vi "Simple Shared Variable and Event Monitor.vi"() -> ()   [LabVIEW 2015]
doc: "This example demonstrates how to build a variable and event monitor using the shared variable Event structure support. \nRefer to the readme.html file in the <b>Project Documentation</b> folder of the project tree for more information about this example."
uses:
  Instance           1 30Saved   Simple Process Monitor .vi
  <vilib>/lvdsc/NI_DSC.lvlib
panel:
  in  "Stop?":bool
  in  "Refresh Variable List":bool
  in  "Delete Variable Button":bool
  in  "Variable List":i32(listbox)=-1
  in  "Delete Process Button":bool
  in  "Deployed Processes":i32(listbox)=-1
  in  "System Events":i32(listbox)=-1
  out "error out":errorcluster
  in  "error in (no error)":errorcluster
  # "LabVIEW DSC Module Example: \nSimple Shared Variable and Event Monitor"
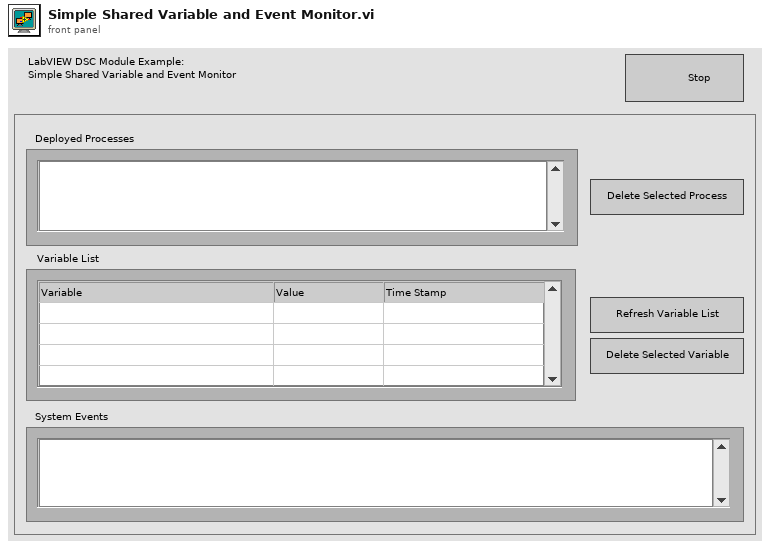
[diagram p1: front panel]
types:
  T1 = enum16{"No Value", "Custom", "Double", "Boolean", "U32", "String", "DBL Array", "I32 Array", "I32", "SGL Array", "SGL", "I8", "U8", "I16", "U16", "I64", "U64", "DBL Waveform", "I16 Waveform", "Boolean Array", "I8 Array", "U8 Array", "I16 Array", "U16 Array", "U32 Array", "I64 Array", "U64 Array", "DBL Waveform Array", "I16 Waveform Array"}
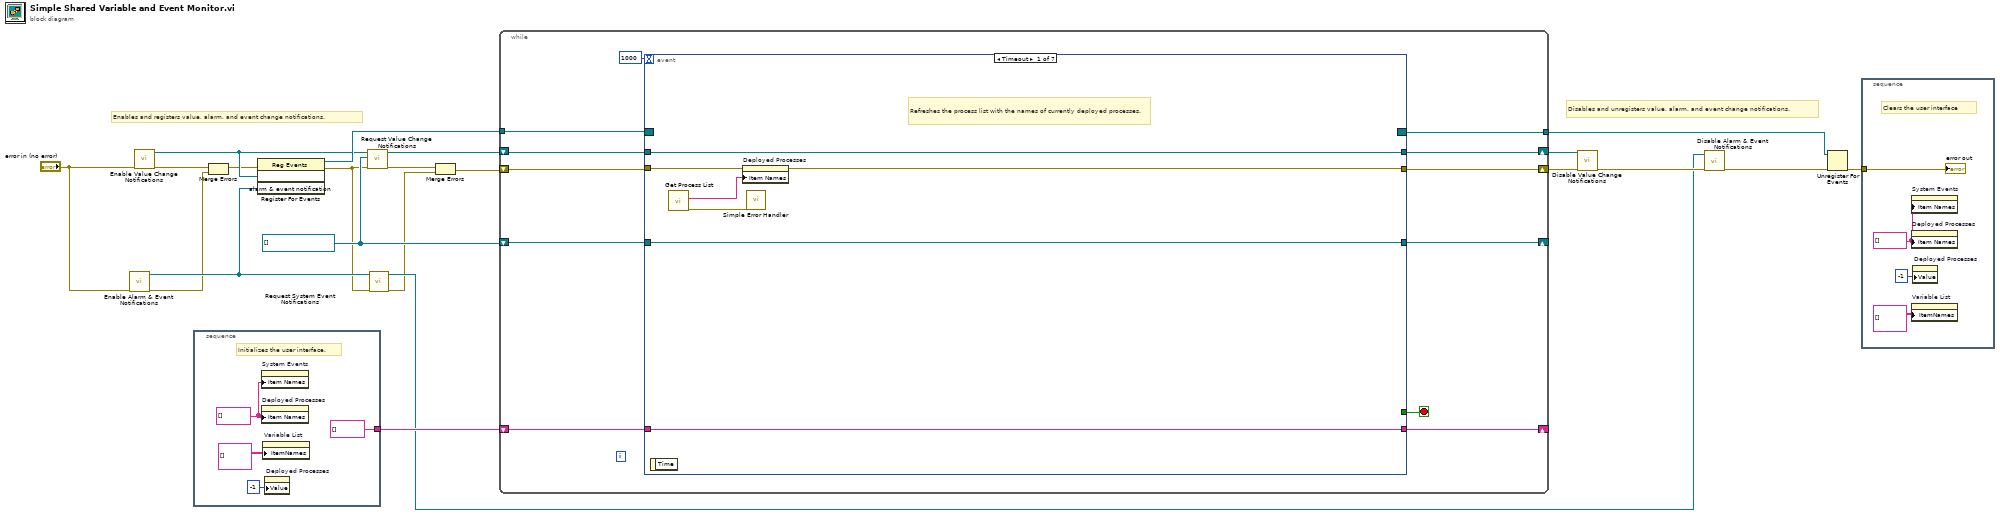
[diagram p0: block diagram]
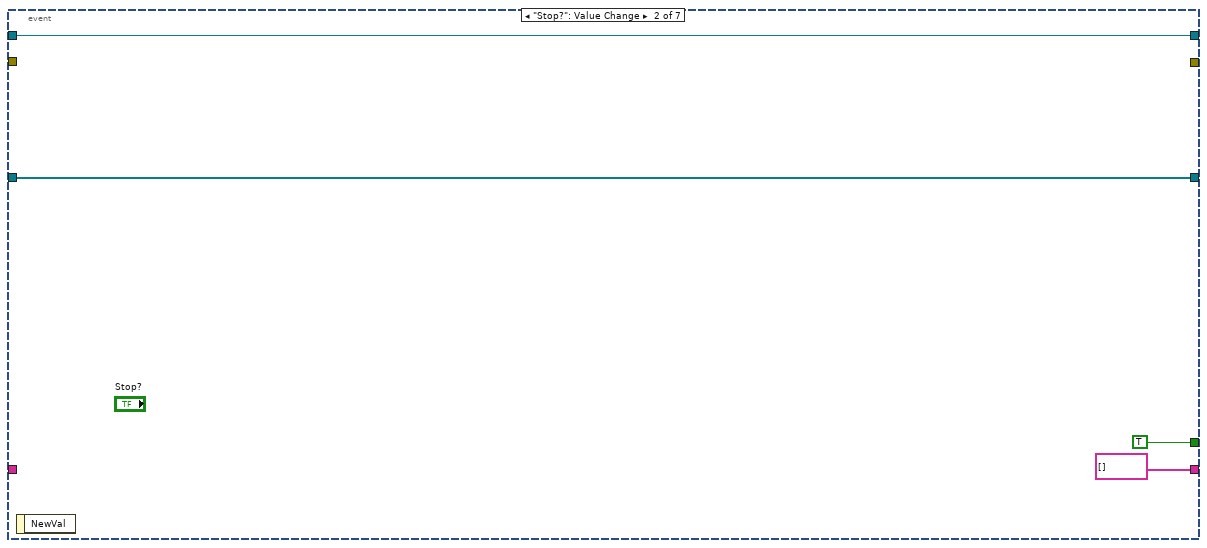
[diagram p2: hidden frame]
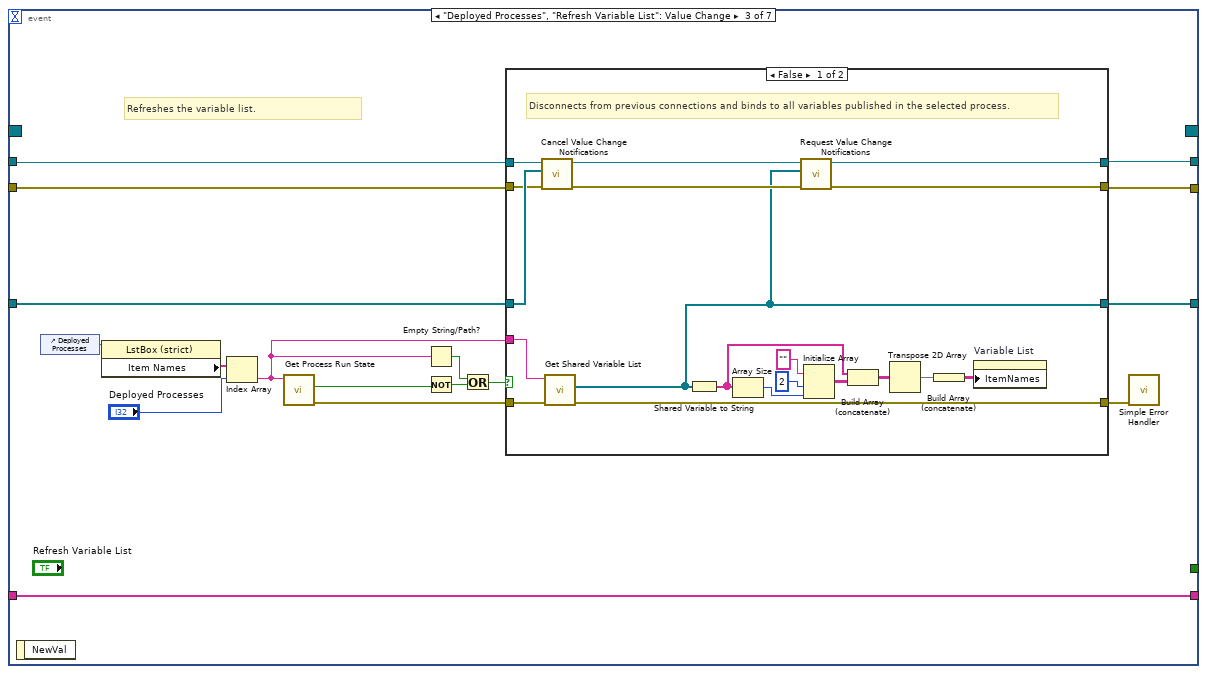
[diagram p3: hidden frame]
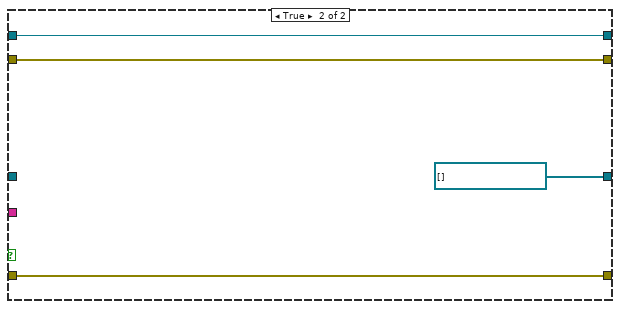
[diagram p4: hidden frame]
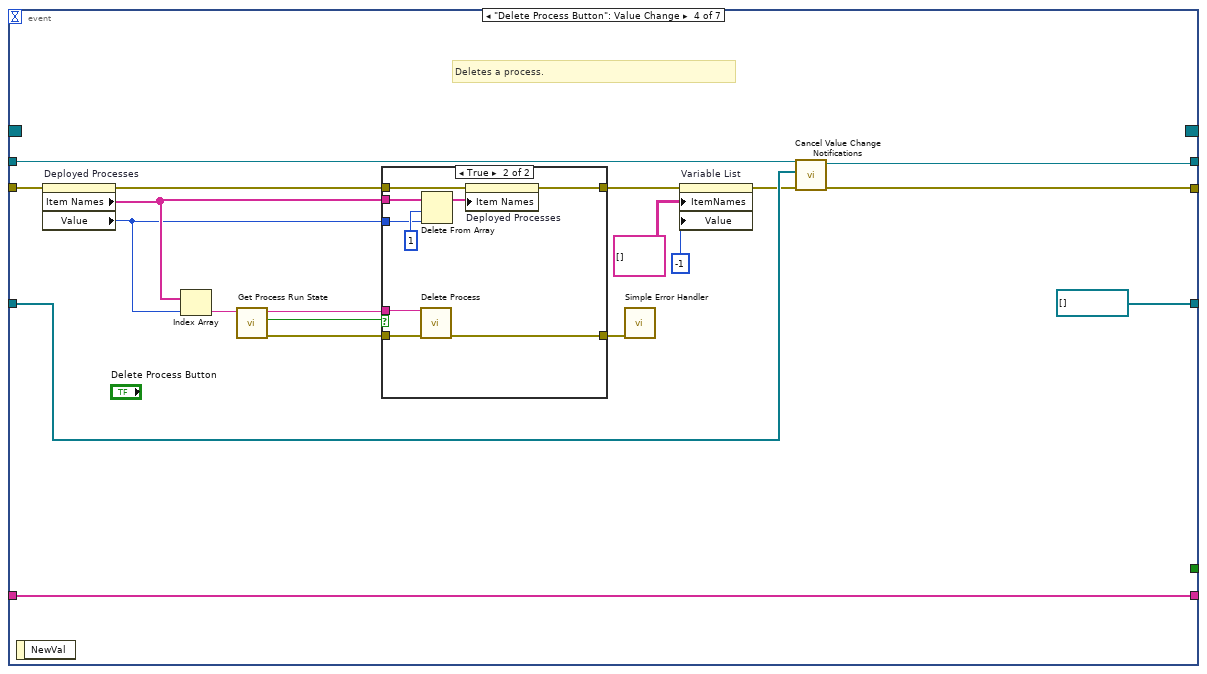
[diagram p5: hidden frame]
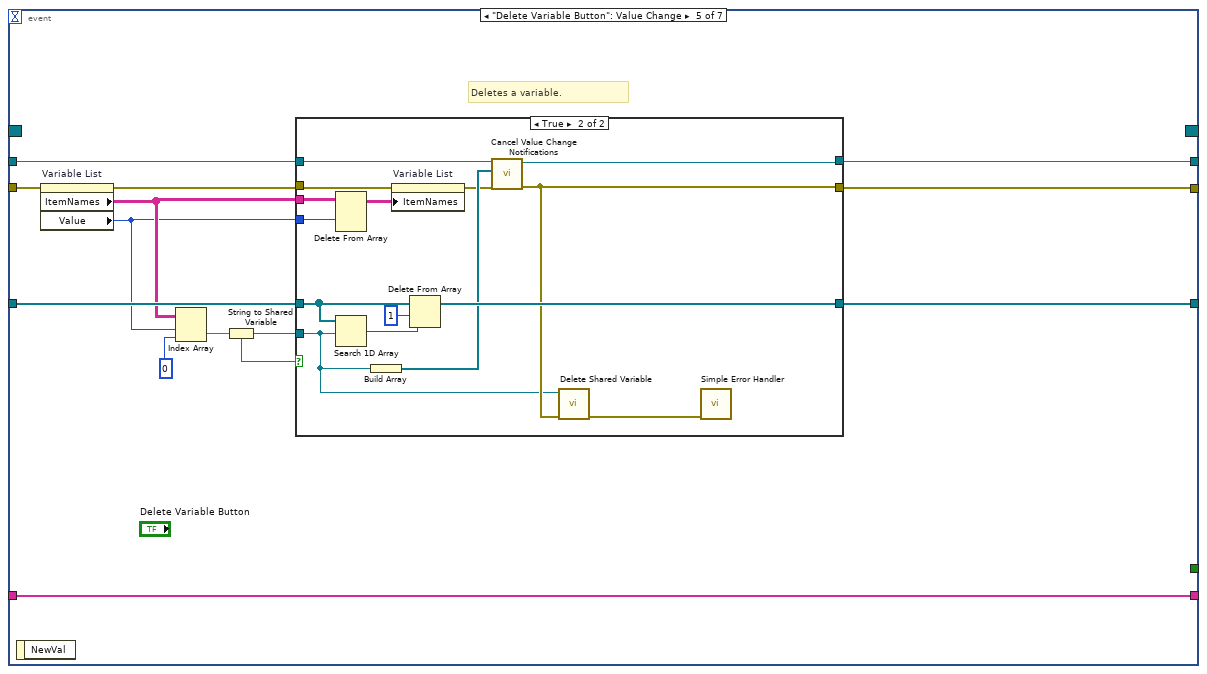
[diagram p7: hidden frame]
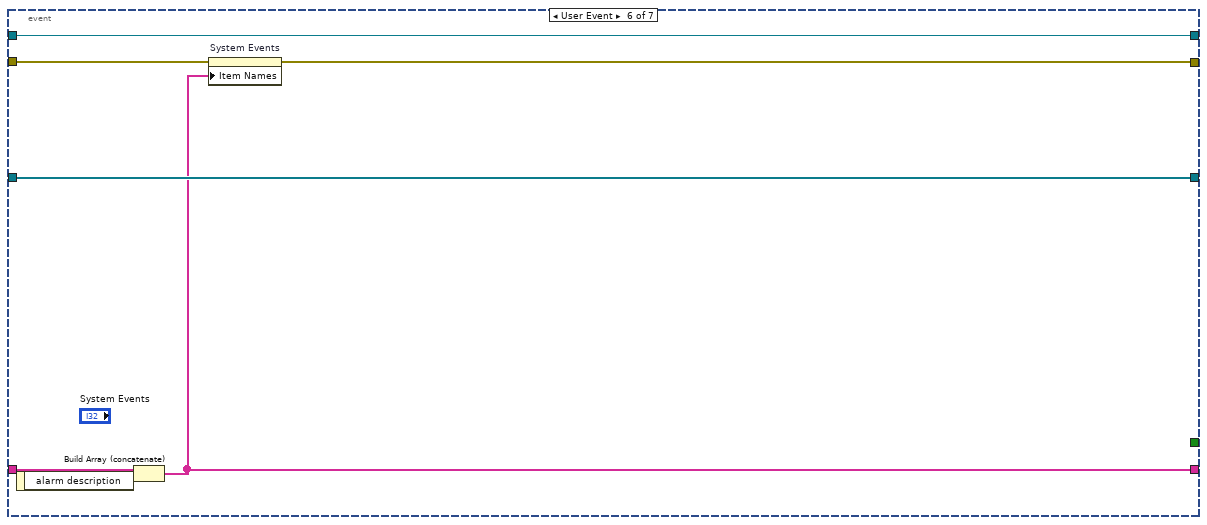
[diagram p9: hidden frame]
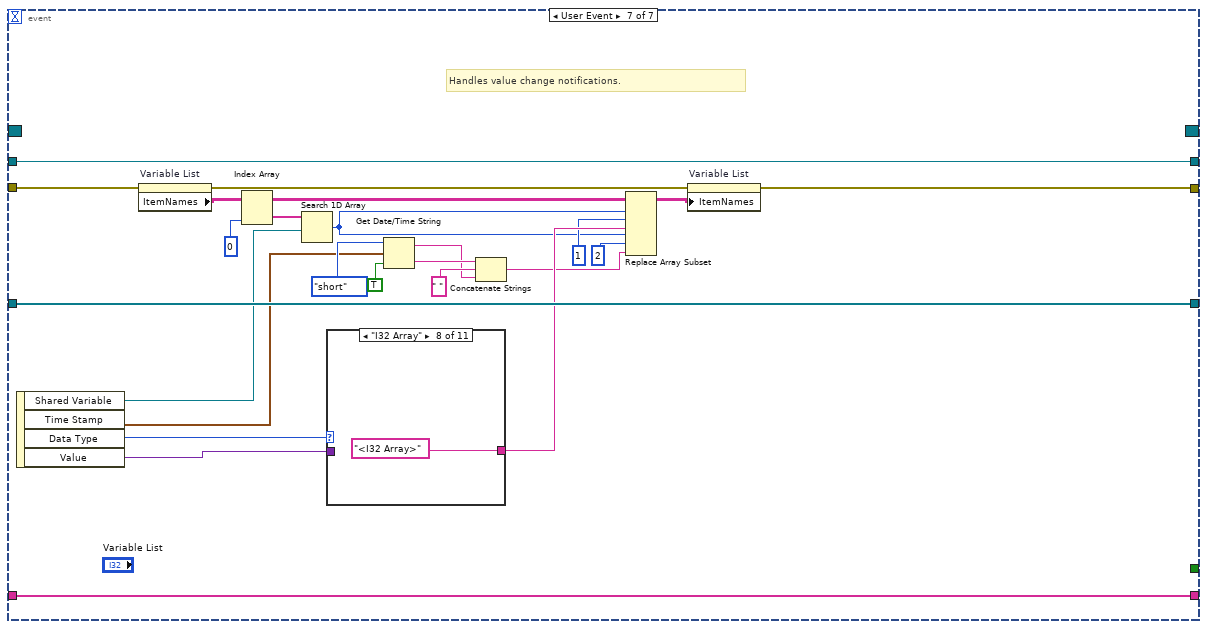
[diagram p10: hidden frame]
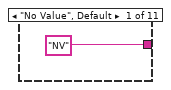
[diagram p11: hidden frame]
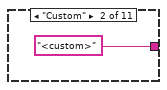
[diagram p12: hidden frame]
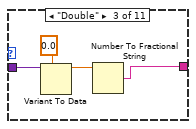
[diagram p13: hidden frame]
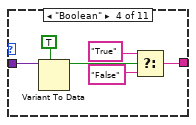
[diagram p14: hidden frame]
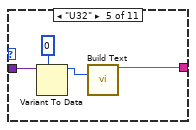
[diagram p15: hidden frame]
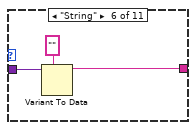
[diagram p16: hidden frame]
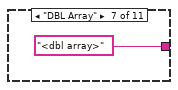
[diagram p17: hidden frame]
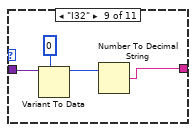
[diagram p18: hidden frame]
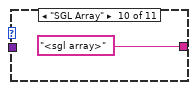
[diagram p19: hidden frame]
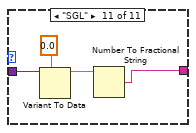
[diagram p20: hidden frame]
diagram:
  w20 = refnum<k21>[] [] ("shared variables")
  # "Disables and unregisters value, alarm, and event change notifications."
  # "Enables and registers value, alarm, and event change notifications."
  n1 = call <vilib>:"Enable Alarm & Event Notifications.vi"("error in (no error)"="error in (no error)") -> ("error out"=w5:errorcluster, "alarm & event notification"=w8:refnum<user-event>)  [unwired: 9 out]
  n2 = call <vilib>:"Enable Value Change Notifications.vi"("error in (no error)"="error in (no error)") -> ("error out"=w7:errorcluster, "shared variable value change notification"=w9:refnum<user-event>)  [unwired: 9 out]
  n3 = stacked-sequence {
    tunnel: [string[] []] -> w17
    frame #0 {
      w23 = string[] [] ("Item Names")
      # "Initializes the user interface."
      n4 = property on="System Events" class="LstBox (strict)"("Item Names"=w23) -> ()  [unwired: 2 in, 2 out]
      n5 = property on="Deployed Processes" class="LstBox (strict)"("Item Names"=w23) -> ()  [unwired: 2 in, 2 out]
      n6 = property on="Variable List" class="MCListbox (strict)"("ItemNames"=string[][] [] ("Item Names")) -> ()  [unwired: 2 in, 2 out]
      n7 = property on="Deployed Processes" class="LstBox (strict)"("Value"=-1 ("Process List")) -> ()  [unwired: 2 in, 2 out]
    }
  }
  n8 = Merge Errors(w7, w5) -> (w6:errorcluster)
  n9 = register-events(error in=w6, w9, w8) -> (reference out=w21:refnum<event-registration>, error out=w4:errorcluster)  [unwired: 1 in]
  n10 = call <vilib>:"Request Value Change Notifications.vi"("error in (no error)"=w4, "shared variables"=w20, "notification refnum"=w9) -> ("error out"=w3:errorcluster, "shared variable value change notification"=w12:refnum<user-event>)  [unwired: 1 in, 6 out]
  n11 = call <vilib>:"Request System Event Notifications.vi"("error in (no error)"=w4, "notification refnum"=w8) -> ("error out"=w2:errorcluster, "alarm & event notification"=w14:refnum<user-event>)  [unwired: 1 in, 7 out]
  n12 = Merge Errors(w3, w2) -> (w1:errorcluster)
  n13 = while {
    tunnel: w21 -> [w36]
    shift-right: [w34] -> _
    shift-left: w17 -> [w35]
    shift-right: [w26] -> _
    shift-left: w20 -> [w31]
    shift-right: [w30] -> w19
    shift-left: w12 -> [w32]
    tunnel: [w29] -> w11
    shift-right: [w28] -> w13
    shift-left: w1 -> [w27]
    stop <- w37 stop-if-true
    n14 = event shown="[0] Timeout" {
      selector: w36 -> [_ _ _ _ _ _ _]
      dyn-events: [_ _ _ _ _ _ _] -> w29
      timeout: 1000 -> [_ _ _ _ _ _ _]
      tunnel: [_ TRUE ("Stop?") _ _ _ _ _] -> w37
      tunnel: w32 -> [w42 w46 w63 w102 w128 w154 w169]
      tunnel: w35 -> [w41 _ w62 w103 w124 w157 w181]
      tunnel: [w41 string[] [] w62 w103 w124 w153 w181] -> w34
      tunnel: w31 -> [w43 w47 w64 w101 w130 w155 w180]
      tunnel: [w43 w47 w59 refnum<k21>[] [] ("shared variables") w129 w155 w180] -> w26
      tunnel: [w42 w46 w50 w100 w125 w154 w169] -> w30
      tunnel: w27 -> [w40 _ w52 w91 w120 w151 w159]
      tunnel: [w39 _ w51 w96 w121 w152 w162] -> w28
      event Timeout {
        # "Refreshes the process list with the names of currently deployed processes."
        n15 = event-data() -> ()  [unwired: 2 out]
        n16 = call <vilib>:"Get Process List.vi"() -> ("error out"=w38:errorcluster, "processes"=w44:string[])  [unwired: 1 in, 9 out]
        n17 = property on="Deployed Processes" class="LstBox (strict)"(error in=w40, "Item Names"=w44) -> (error out=w39:errorcluster)  [unwired: 1 in, 1 out]
        n18 = call <vilib>:"Simple Error Handler.vi"("error in (no error)"=w38) -> ()  [unwired: 4 in, 5 out]
      }
      event "Stop?": Value Change {
        n19 = event-data() -> ()  [unwired: 2 out]
      }
      event "Deployed Processes", "Refresh Variable List": Value Change {
        # "Refreshes the variable list."
        n20 = event-data() -> ()  [unwired: 2 out]
        n21 = control-ref of="Deployed Processes"() -> (w61:refnum<vi>)
        n22 = property class="LstBox (strict)"(reference=w61) -> ("Item Names"=w65:string[])  [unwired: 1 in, 2 out]
        n23 = Index Array(array=w65, index="Deployed Processes") -> (element=w58:string)
        n24 = call <vilib>:"Get Process Run State.vi"("process name"=w58) -> ("error out"=w53:errorcluster, "exists?"=w56:bool)  [unwired: 1 in, 8 out]
        n25 = Empty String/Path?(string/path=w58) -> (empty?=w57:bool)
        n26 = Not(x=w56) -> (.not. x?=w54:bool)
        n27 = Or(x=w57, y=w54) -> (x .or. y?=w55:bool)
        n28 = case shown="False" w55 {
          tunnel: w58 -> [w84 _]
          tunnel: w64 -> [w81 _]
          tunnel: w63 -> [w80 w87]
          tunnel: [w73 w87] -> w50
          tunnel: [w69 refnum<k21>[] [] ("shared variables")] -> w59
          tunnel: w53 -> [w70 w85]
          tunnel: w52 -> [w68 w86]
          tunnel: [w67 w86] -> w51
          tunnel: [w66 w85] -> w49
          frame False {
            # "Disconnects from previous connections and binds to all variables published in the selected process."
            n29 = call <vilib>:"Cancel Value Change Notifications.vi"("error in (no error)"=w68, "shared variables"=w81, "notification refnum"=w80) -> ("error out"=w82:errorcluster, "shared variable value change notification"=w83:refnum<user-event>)  [unwired: 7 out]
            n30 = call <vilib>:"Get Shared Variable List.vi"("error in (no error)"=w70, "process name"=w84) -> ("error out"=w66:errorcluster, "shared variables"=w69:refnum<k21>[])  [unwired: 8 out]
            n31 = Shared Variable to String(1:w69) -> (0:w72:string[])
            n32 = Array Size(array=w72) -> (size(s)=w74:i32)
            n33 = call <vilib>:"Request Value Change Notifications.vi"("error in (no error)"=w82, "shared variables"=w69, "notification refnum"=w83) -> ("error out"=w67:errorcluster, "shared variable value change notification"=w73:refnum<user-event>)  [unwired: 1 in, 6 out]
            n34 = Initialize Array("", 2 ("dimension size"), w74) -> (w76:string[][])
            n35 = Build Array (concatenate)(w72, w76) -> (w75:string[][])
            n36 = Transpose 2D Array(2D array=w75) -> (transposed array=w79:string[][])
            n37 = Build Array (concatenate)(w79) -> (w78:string[][])
            n38 = property on="Variable List" class="MCListbox (strict)"("ItemNames"=w78) -> ()  [unwired: 2 in, 2 out]
          }
          frame True {
          }
        }
        n39 = call <vilib>:"Simple Error Handler.vi"("error in (no error)"=w49) -> ()  [unwired: 4 in, 5 out]
      }
      event "Delete Process Button": Value Change {
        # "Deletes a process."
        n40 = event-data() -> ()  [unwired: 2 out]
        n41 = property on="Deployed Processes" class="LstBox (strict)"(error in=w91) -> (error out=w89:errorcluster, "Item Names"=w98:string[], "Value"=w92:i32)  [unwired: 1 in, 1 out]
        n42 = Index Array(array=w98, index=w92) -> (element=w106:string)
        n43 = call <vilib>:"Get Process Run State.vi"("process name"=w106) -> ("error out"=w97:errorcluster, "exists?"=w105:bool, "process name out"=w107:string)  [unwired: 1 in, 7 out]
        n44 = case shown="True" w105 {
          tunnel: w97 -> [w109 w112]
          tunnel: w107 -> [_ w118]
          tunnel: w98 -> [_ w117]
          tunnel: w92 -> [_ w115]
          tunnel: [w109 w113] -> w94
          tunnel: w89 -> [w108 w111]
          tunnel: [w108 w110] -> w93
          frame False {
          }
          frame True {
            n45 = call <vilib>:"Delete Process.vi"("error in (no error)"=w112, "process name"=w118) -> ("error out"=w113:errorcluster)  [unwired: 9 out]
            n46 = Delete From Array(array=w117, length=1, index=w115) -> (array with subset deleted=w114:string[])  [unwired: 1 out]
            n47 = property on="Deployed Processes" class="LstBox (strict)"(error in=w111, "Item Names"=w114) -> (error out=w110:errorcluster)  [unwired: 1 in, 1 out]
          }
        }
        n48 = call <vilib>:"Simple Error Handler.vi"("error in (no error)"=w94) -> ()  [unwired: 4 in, 5 out]
        n49 = property on="Variable List" class="MCListbox (strict)"(error in=w93, "ItemNames"=string[][] [] ("Item Names"), "Value"=-1 ("Process List")) -> (error out=w95:errorcluster)  [unwired: 1 in, 1 out]
        n50 = call <vilib>:"Cancel Value Change Notifications.vi"("error in (no error)"=w95, "shared variables"=w101, "notification refnum"=w102) -> ("error out"=w96:errorcluster, "shared variable value change notification"=w100:refnum<user-event>)  [unwired: 7 out]
      }
      event "Delete Variable Button": Value Change {
        # "Deletes a variable."
        n51 = event-data() -> ()  [unwired: 2 out]
        n52 = property on="Variable List" class="MCListbox (strict)"(error in=w120) -> (error out=w126:errorcluster, "ItemNames"=w127:string[][], "Value"=w119:i32)  [unwired: 1 in, 1 out]
        n53 = Index Array(array=w127, index (row)=w119, index (col)=0 ("disabled index (col)")) -> (element=w132:string)
        n54 = String to Shared Variable(0:w132) -> (1:w122:bool, 2:w123:refnum<k21>)
        n55 = case shown="True" w122 {
          tunnel: w130 -> [w134 w150]
          tunnel: [w134 w149] -> w129
          tunnel: w128 -> [w135 w146]
          tunnel: w127 -> [_ w144]
          tunnel: w119 -> [_ w143]
          tunnel: w126 -> [w133 w141]
          tunnel: [w135 w140] -> w125
          tunnel: w123 -> [_ w136]
          tunnel: [w133 w137] -> w121
          frame False {
          }
          frame True {
            n56 = Delete From Array(array=w144, index (row)=w143) -> (array with subset deleted=w142:string[][])  [unwired: 2 in, 1 out]
            n57 = Search 1D Array(1D array=w150, element=w136) -> (index of element=w148:i32)  [unwired: 1 out]
            n58 = Build Array(w136) -> (w145:refnum<k21>[])
            n59 = property on="Variable List" class="MCListbox (strict)"(error in=w141, "ItemNames"=w142) -> (error out=w138:errorcluster)  [unwired: 1 in, 1 out]
            n60 = Delete From Array(array=w150, length=1, index=w148) -> (array with subset deleted=w149:refnum<k21>[])  [unwired: 1 out]
            n61 = call <vilib>:"Cancel Value Change Notifications.vi"("error in (no error)"=w138, "shared variables"=w145, "notification refnum"=w146) -> ("error out"=w137:errorcluster, "shared variable value change notification"=w140:refnum<user-event>)  [unwired: 7 out]
            n62 = call <vilib>:"Delete Shared Variable.vi"("error in (no error)"=w137, "shared variable"=w136) -> ("error out"=w139:errorcluster)  [unwired: 9 out]
            n63 = call <vilib>:"Simple Error Handler.vi"("error in (no error)"=w139) -> ()  [unwired: 4 in, 5 out]
          }
        }
      }
      event User Event {
        n64 = event-data() -> ("alarm description"=w156:string)  [unwired: 1 out]
        n65 = Build Array (concatenate)(w157, w156) -> (w153:string[])
        n66 = property on="System Events" class="LstBox (strict)"(error in=w151, "Item Names"=w153) -> (error out=w152:errorcluster)  [unwired: 1 in, 1 out]
      }
      event User Event {
        # "Handles value change notifications."
        n67 = event-data() -> ("Shared Variable"=w163:refnum<k21>, "Time Stamp"=w168:timestamp, "Data Type"=w160:T1, "Value"=w161:variant)  [unwired: 1 out]
        n68 = property on="Variable List" class="MCListbox (strict)"(error in=w159) -> (error out=w164:errorcluster, "ItemNames"=w165:string[][])  [unwired: 1 in, 1 out]
        n69 = Index Array(array=w165, index (col)=0 ("disabled index (col)")) -> (element=w178:string[])  [unwired: 1 in]
        n70 = Search 1D Array(1D array=w178, element=w163) -> (index of element=w166:i32)  [unwired: 1 out]
        n71 = case shown="\"I32 Array\"" w160 {
          tunnel: w161 -> [_ _ w187 w193 w197 w200 _ _ w206 _ w208]
          tunnel: ["NV" "<custom>" w184 w188 w194 w198 "<dbl array>" ("Result") "<I32 Array>" ("Result") w203 "<sgl array>" ("Result") w209] -> w177
          frame "No Value", Default {
          }
          frame "Custom" {
          }
          frame "Double" {
            n72 = Variant To Data(type=0.0 ("disabled index (col)"), Variant=w187) -> (data=w185:dbl)  [unwired: 1 in, 1 out]
            n73 = Number To Fractional String(number=w185) -> (F-format string=w184:string)  [unwired: 3 out]
          }
          frame "Boolean" {
            n74 = Variant To Data(type=TRUE, Variant=w193) -> (data=w191:bool)  [unwired: 1 in, 1 out]
            n75 = Select(t="True", s=w191, f="False") -> (s? t:f=w188:string)
          }
          frame "U32" {
            n76 = Variant To Data(type=u32 0, Variant=w197) -> (data=w195:u32)  [unwired: 1 in, 1 out]
            n77 = call "Build Text"("bitarray"=w195) -> ("Result"=w194:string)  [unwired: 2 in, 12 out]
          }
          frame "String" {
            n78 = Variant To Data(type="", Variant=w200) -> (data=w198:string)  [unwired: 1 in, 1 out]
          }
          frame "DBL Array" {
          }
          frame "I32 Array" {
          }
          frame "I32" {
            n79 = Variant To Data(type=0 ("disabled index (row)"), Variant=w206) -> (data=w204:i32)  [unwired: 1 in, 1 out]
            n80 = Number To Decimal String(number=w204) -> (decimal integer string=w203:string)  [unwired: 1 out]
          }
          frame "SGL Array" {
          }
          frame "SGL" {
            n81 = Variant To Data(type=sgl 0.0 ("disabled index (col)"), Variant=w208) -> (data=w210:sgl)  [unwired: 1 in, 1 out]
            n82 = Number To Fractional String(number=w210) -> (F-format string=w209:string)  [unwired: 3 out]
          }
        }
        n83 = Get Date/Time String(date format (0)=enum16{"short", "long", "abbreviated"}."short", seconds (now)=w168, want seconds? (F)=TRUE) -> (date string=w158:string, time string=w175:string)
        n84 = Concatenate Strings(w175, " " ("string"), w158) -> (w172:string)
        n85 = Replace Array Subset(array=w165, new element #1=w177, index (row) #1=w166, index (col) #1=1 ("disabled index (row)"), new element #2=w172, index (row) #2=w166, index (col) #2=2 ("index (col)")) -> (w167:string[][])
        n86 = property on="Variable List" class="MCListbox (strict)"(error in=w164, "ItemNames"=w167) -> (error out=w162:errorcluster)  [unwired: 1 in, 1 out]
      }
    }
  }
  n87 = call <vilib>:"Disable Value Change Notifications.vi"("error in (no error)"=w13, "notification refnum"=w19) -> ("error out"=w16:errorcluster)  [unwired: 9 out]
  n88 = call <vilib>:"Disable Alarm & Event Notifications.vi"("error in (no error)"=w16, "notification refnum"=w14) -> ("error out"=w15:errorcluster)  [unwired: 9 in]
  n89 = Unregister For Events(event registration refnum=w11, error in=w15) -> (error out=w18:errorcluster)
  n90 = stacked-sequence {
    tunnel: w18 -> [w212]
    frame #0 {
      w213 = string[] [] ("Item Names")
      # "Clears the user interface"
      n91 = property on="System Events" class="LstBox (strict)"("Item Names"=w213) -> ()  [unwired: 2 in, 2 out]
      n92 = property on="Deployed Processes" class="LstBox (strict)"("Item Names"=w213) -> ()  [unwired: 2 in, 2 out]
      n93 = property on="Variable List" class="MCListbox (strict)"("ItemNames"=string[][] [] ("Item Names")) -> ()  [unwired: 2 in, 2 out]
      n94 = property on="Deployed Processes" class="LstBox (strict)"("Value"=-1 ("Process List")) -> ()  [unwired: 2 in, 2 out]
      "error out" <- w212
    }
  }
